vi "StateMachineP7.vi"() -> ()   [LabVIEW 2013]
doc: "Use this template to build a simple state machine design pattern. Each state executes code and determines which state to transition to."
uses:
  StatemMachineLV7/controls/State.ctl
panel:
  out "Alarm Indicator":bool
  out "Alarm Events":dbl
  out "Waveform Chart":dbl(graph)
  out "Temp. Values":dbl
  in  "?":bool
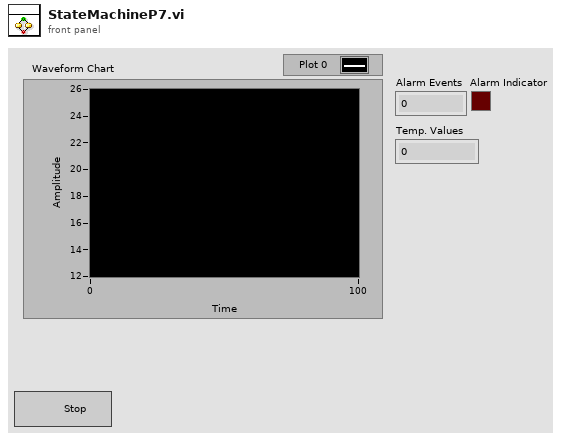
[diagram p1: front panel]
types:
  T1 = typedef "State.ctl" = enum16{"Acquire", "Analyze", "Alarm"}
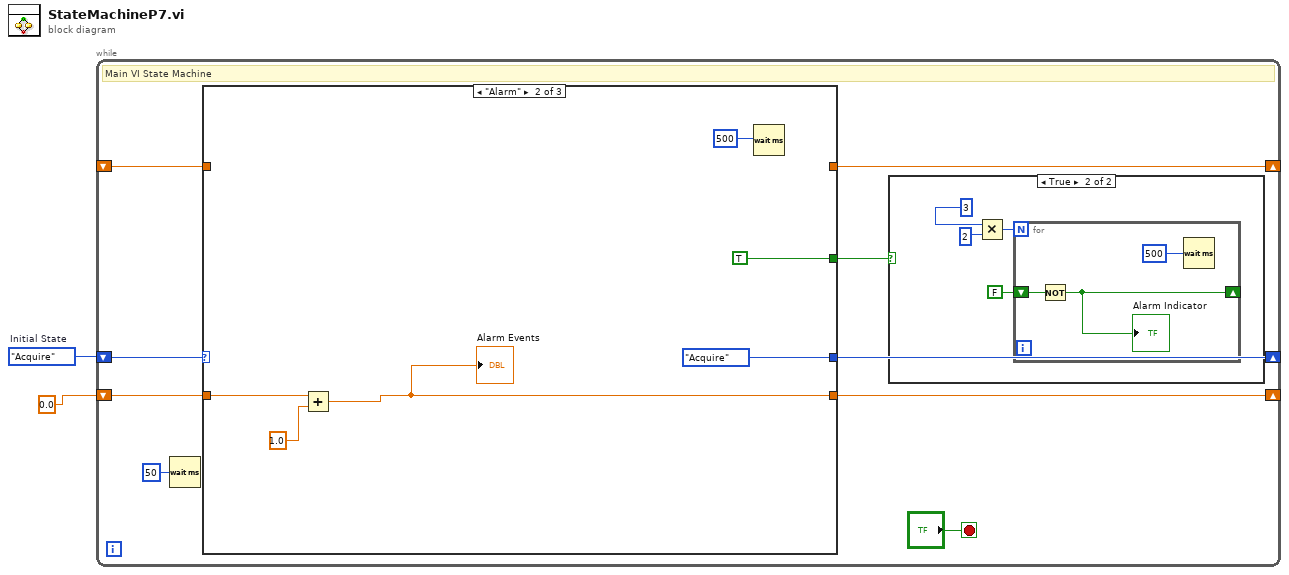
[diagram p0: block diagram]
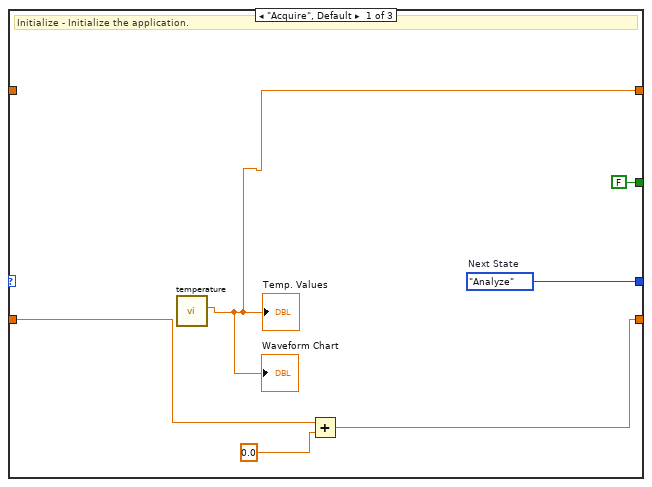
[diagram p3: hidden frame]
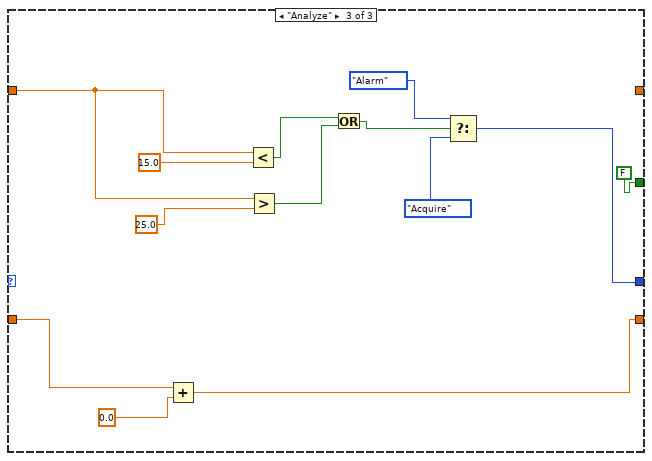
[diagram p4: hidden frame]
diagram:
  w2 = State."Acquire"  # Initial State
  n1 = while {
    shift-right: [w10] -> _
    shift-left: w2 -> [w11]
    shift-right: [w7] -> _
    shift-left: _ -> [w6]
    shift-right: [w5] -> _
    shift-left: 0.0 ("x") -> [w4]
    stop <- "?" stop-if-true
    # "Main VI State Machine"
    n2 = Wait (ms)(milliseconds to wait=u32 50) -> ()  [unwired: 1 out]
    n3 = case shown="\"Alarm\"" w11 {
      tunnel: [w24 State."Acquire" w36] -> w10
      tunnel: [w23 _ _] -> w7
      tunnel: w6 -> [_ _ w37]
      tunnel: [w20 w28 w33] -> w5
      tunnel: w4 -> [w21 w27 w34]
      tunnel: [FALSE ("Run") TRUE FALSE ("Run")] -> w3
      frame "Acquire", Default {
        w24 = State."Analyze"  # Next State
        # "Initialize - Initialize the application."
        n4 = call "temperature.vi"() -> ("Temperature (C)"=w23:dbl)  [unwired: 10 in, 1 out]
        "Temp. Values" <- w23
        "Waveform Chart" <- w23
        n5 = Add(x=w21, y=0.0) -> (x+y=w20:dbl)
      }
      frame "Alarm" {
        n6 = Add(x=w27, y=1.0) -> (x+y=w28:dbl)
        "Alarm Events" <- w28
        n7 = Wait (ms)(milliseconds to wait=u32 500) -> ()  [unwired: 1 out]
      }
      frame "Analyze" {
        n8 = Add(x=w34, y=0.0) -> (x+y=w33:dbl)
        n9 = Less?(x=w37, y=15.0) -> (x < y?=w40:bool)
        n10 = Greater?(x=w37, y=25.0) -> (0:w41:bool)
        n11 = Or(x=w40, y=w41) -> (x .or. y?=w32:bool)
        n12 = Select(t=State."Alarm" ("Next State"), s=w32, f=State."Acquire" ("Next State")) -> (s? t:f=w36:T1)
      }
    }
    n13 = case shown="True" w3 {
      frame False {
      }
      frame True {
        n14 = Multiply(x=3, y=2) -> (x*y=w15:i32)
        n15 = for {
          N: w15 -> [_]
          shift-right: [w16] -> _
          shift-left: FALSE -> [w17]
          n16 = Not(x=w17) -> (.not. x?=w16:bool)
          "Alarm Indicator" <- w16
          n17 = Wait (ms)(milliseconds to wait=u32 500) -> ()  [unwired: 1 out]
        }
      }
    }
  }
